vi "Config Reference Mask.vi"(8 "error in":errorcluster, 9 "Loss Mask (on)":enum16{"off", "on"}(ring)=enum."on", 10 "Capacitance Mask (on)":enum16{"off", "on"}(ring)=enum."on", 11 "VISA resource name":refnum<visa-resource-name>) -> (0 "error out":errorcluster, 3 "VISA resource name out":refnum<visa-resource-name>)   [LabVIEW 2019, in "Andeen-Hagerling 2700(400 firmware).lvlib"]
doc: "Enables the reporting of reference results for capacitance and / or loss."
uses:
  Andeen-Hagerling 2700(400 firmware).lvlib
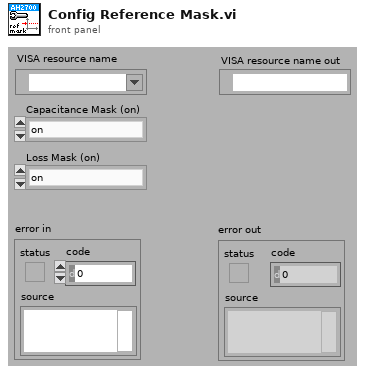
[diagram p1: front panel]
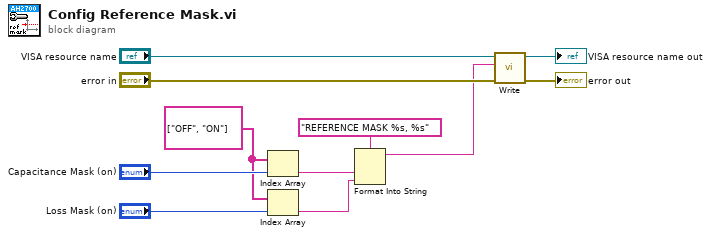
[diagram p0: block diagram]
diagram:
  w3 = string[] ["OFF", "ON"]
  n1 = Index Array(array=w3, index="Capacitance Mask (on)") -> (element=w2:string)
  n2 = Index Array(array=w3, index="Loss Mask (on)") -> (element=w1:string)
  n3 = Format Into String(format string="REFERENCE MASK %s, %s", w2, w1) -> (resulting string=w6:string)  [unwired: 2 in, 1 out]
  n4 = call "Write.vi"("error in"="error in", "command"=w6, "VISA resource name"="VISA resource name") -> ("error out"=→"error out":errorcluster, "VISA resource name out"=→"VISA resource name out":refnum<visa-resource-name>)  [unwired: 7 in]
